vi "Create Decision Event.vi"(10 "Boolean":bool, 11 "User Event in":refnum<user-event>) -> ()   [LabVIEW 2011]
uses:
  DecisionCluster_typdef.ctl
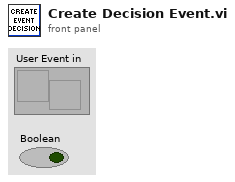
[diagram p1: front panel]
types:
  T1 = typedef "DecisionCluster_typdef.ctl" = cluster{"vi path":path, "Message":string}
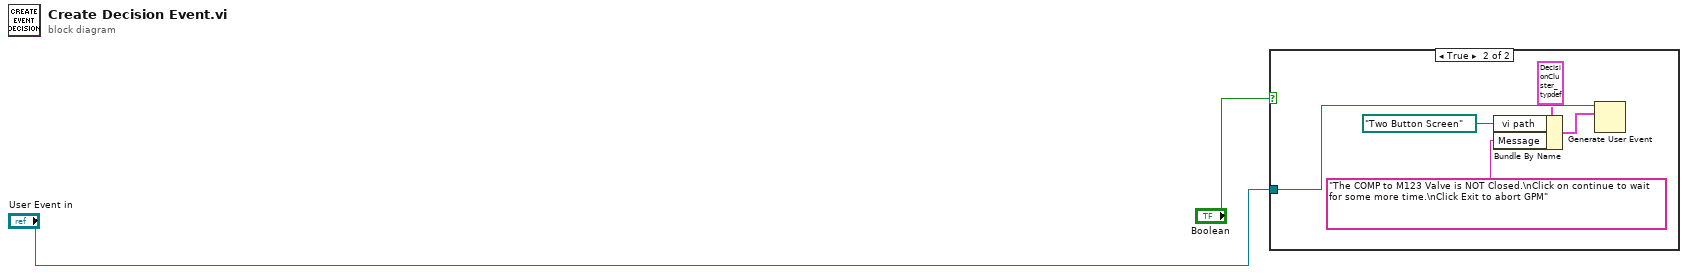
[diagram p0: block diagram]
diagram:
  n1 = case shown="True" "Boolean" {
    tunnel: "User Event in" -> [_ w7]
    frame False {
    }
    frame True {
      n2 = Bundle By Name(cluster=T1 {"vi path"=path "Dummy.vi", "Message"=""}, "vi path"=path "Two Button Screen" ("event data"), "Message"="The COMP to M123 Valve is NOT Closed.\nClick on continue to wait for some more time.\nClick Exit to abort GPM" ("message")) -> (w3:T1)
      n3 = Generate User Event(user event=w7, event data cluster=w3) -> ()  [unwired: 1 in, 2 out]
    }
  }
